vi "_TEST Drivers.vi"(4 "error in (no error)":errorcluster) -> (0 "error out":errorcluster)   [LabVIEW 2011]
uses:
  Driver Record.ctl
  Driver Table Fields.ctl
panel:
  out "Driver Record":T1
  out "Driver Records":T1[](array[typedef])
  in  "Sort by Field (Name)":T2
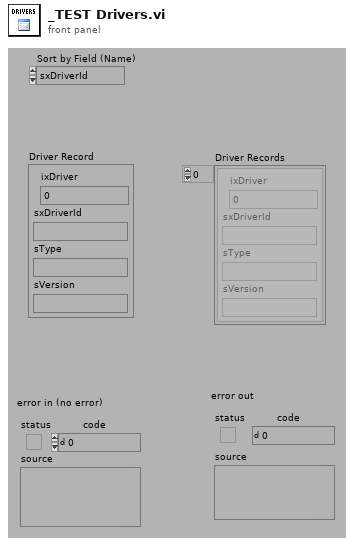
[diagram p1: front panel]
types:
  T1 = typedef "Driver Record.ctl" = cluster{"ixDriver":i32, "sxDriverId":string, "sType":string, "sVersion":string}
  T2 = typedef "Driver Table Fields.ctl" = enum16{"sxDriverId", "sType", "sVersion", "ixDriver"}
  T3 = typedef "Connection Refnum.ctl" = cluster{"Environment Handle":i32, "Connection Handle":i32}
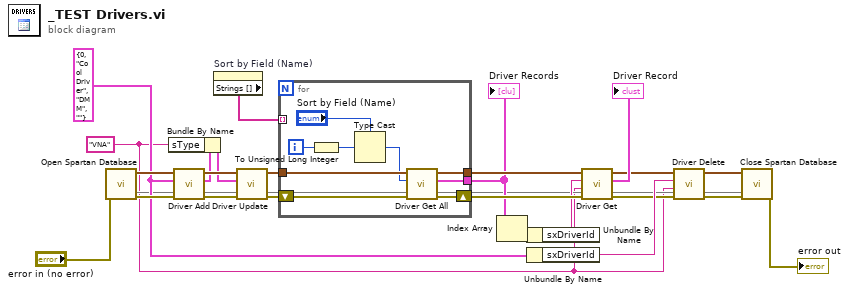
[diagram p0: block diagram]
diagram:
  w1 = "VNA" ("DriverType")
  w15 = T1 {"ixDriver"=0, "sxDriverId"="Cool Driver", "sType"="DMM", "sVersion"=""} ("Driver Record")
  n1 = call "Open Spartan Database.vi"("error in (no error)"="error in (no error)") -> ("error out"=w25:errorcluster, "Connection Refnum"=w24:T3, 4:w10)  [unwired: 1 in, 7 out]
  n2 = call "Driver Add.vi"("error in (no error)"=w25, "Driver Record"=w15, "Connection Refnum"=w24) -> ("error out"=w5:errorcluster, "New Driver Record"=w3:T1, "Connection Refnum"=w7:T3)  [unwired: 6 out]
  n3 = Bundle By Name(cluster=w3, "sType"=w1) -> (w2:T1)
  n4 = property on="Sort by Field (Name)" class="Enum (strict)"() -> ("Strings []"=w23:string[])  [unwired: 2 in, 2 out]
  n5 = call "Driver Update.vi"("error in (no error)"=w5, "Driver Record"=w2, "Connection Refnum"=w7) -> ("error out"=w4:errorcluster, "Connection Refnum"=w6:T3)  [unwired: 7 out]
  n6 = for {
    shift-right: [w28] -> w21
    shift-left: w4 -> [w29]
    tunnel: w6 -> [w34]
    tunnel: w23 -> [_] mode=indexing
    tunnel: [w27] -> w22
    tunnel: [w26] -> w20
    i -> [w32]
    n7 = To Unsigned Long Integer(number=w32) -> (unsigned 32bit integer=w31:u32)
    n8 = Type Cast(type="Sort by Field (Name)", x=w31) -> (*(type *) &x=w30:T2)
    n9 = call "Driver Get All.vi"("error in (no error)"=w29, "Sort by (sxDriverId)"=w30, "Connection Refnum"=w34) -> ("error out"=w28:errorcluster, "Drivers"=w26:T1[], "Connection Refnum"=w27:T3)  [unwired: 1 in, 5 out]
  }
  "Driver Records" <- w20
  n10 = Index Array(array=w20) -> (element=w19:T1)  [unwired: 1 in]
  n11 = Unbundle By Name(w19) -> ("sxDriverId"=w18:string)
  n12 = Unbundle By Name(w15) -> ("sxDriverId"=w14:string)
  n13 = call "Driver Get.vi"("error in (no error)"=w21, "sType"=w1, "sxDriverId"=w18, "Connection Refnum"=w22) -> ("error out"=w13:errorcluster, "Driver Record"=→"Driver Record":T1, "Connection Refnum"=w16:T3)  [unwired: 5 out]
  n14 = call "Driver Delete.vi"("error in (no error)"=w13, "sType"=w1, "sxDriverId"=w14, "Connection Refnum"=w16) -> ("error out"=w11:errorcluster, "Connection Refnum"=w12:T3)  [unwired: 6 out]
  n15 = call "Close Spartan Database.vi"("Force Close? (f)"=w10, "error in (no error)"=w11, "Connection Refnum"=w12) -> ("error out"=→"error out":errorcluster)  [unwired: 1 in, 7 out]
